vi "_Remote Prepare Run Data.vi"(4 "Ramp Parameters":T6[](array[typedef]), 5 "StepMass":dbl, 6 "# of Cycles":i32, 7 "StartMass":dbl, 8 "error in":errorcluster, 9 "Steps":i32, 10 "Pause (ms)":dbl, 11 "Dwell (ms)":dbl) -> (0 "error out":errorcluster, 3 "AcqMethod":T1[](array[typedef]) {"ScanType" format="%#.6g"; "Mass Range"."Res" items=["High/High", "Medium/Medium", "Low/Low", "High/Medium", "High/Low", "Medium/High", "Medium/Low", "Low/High", "Low/Medium"]})   [LabVIEW 2015]
uses:
  Type/_Ramp Parameter.ctl
  Type/_XML Expt.ctl
  Type/_XML Lens.ctl
  Type/_Mass Range Property.ctl
  Type/_Mass Range Parameters.ctl
  Type/_RT Res Type.ctl
  Type/_RT Parameter.ctl
  Type/_RT Active Ch.ctl
  Type/_RT Expt.ctl
  Type/_Run Mode.ctl
  Type/_RT Mass Range.ctl
  Type/_RT Command.ctl
  Configuration/_Global Configuration.vi
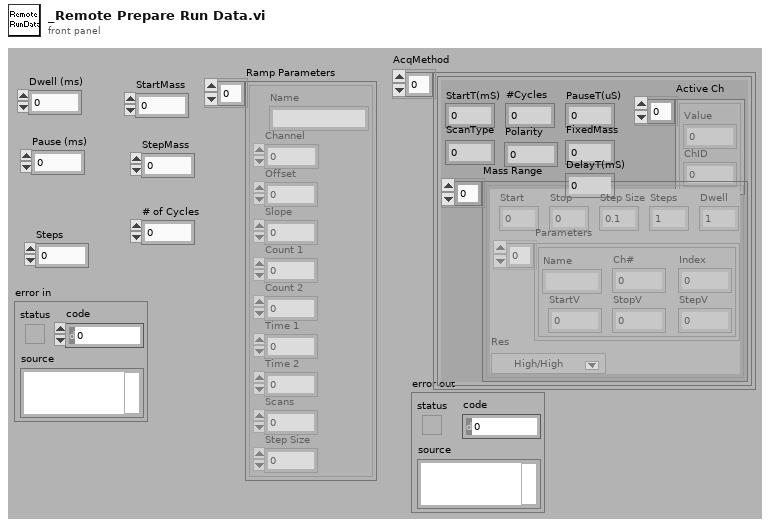
[diagram p1: front panel]
types:
  T1 = typedef "_XML Expt.ctl" = cluster{"StartT(mS)":i32, "#Cycles":i32, "PauseT(uS)":i32, "ScanType":i32, "Polarity":u8, "FixedMass":dbl, "DelayT(mS)":i32, "Active Ch":T2[], "Mass Range":T3[]}
  T2 = typedef "_XML Lens.ctl" = cluster{"Value":dbl, "ChID":u8}
  T3 = typedef "_Mass Range Property.ctl" = cluster{"Start":dbl, "Stop":dbl, "Step Size":dbl, "Steps":i32, "Dwell":dbl, "Parameters":T4[], "Res":T5}
  T4 = typedef "_Mass Range Parameters.ctl" = cluster{"Name":string, "Ch#":u8, "StartV":dbl, "StopV":dbl, "StepV":dbl, "Index":u8}
  T5 = typedef "_RT Res Type.ctl" = u16
  T6 = typedef "_Ramp Parameter.ctl" = cluster{"Name":string, "Channel":u8, "Offset":dbl, "Slope":dbl, "Count 1":dbl, "Count 2":dbl, "Time 1":dbl, "Time 2":dbl, "Scans":i32, "Step Size":dbl}
  T7 = typedef "_RT Command.ctl" = enum16{"xml Start Run", "xml Start Actual Run", "xml Stop Run", "xml Runtime Update", "xml Get Status", "xml Get Table", "xml Set Table", "xml Get Configuration", "xml System Status", "xml Set LC Input Logic", "xml Get Data", "xml Get Info", "Start", "StartActualRun", "Stop", "Runtime Update", "Get Data", "Get Info", "Get Status", "Get Param", "Get Config", "Get Table", "Read ADC", "Set Oscillator", "Update Config", "Update Table", "Set All Pol", "Set Pol and DC", "Set Max Mass", "Toggle RP", "Toggle EL", "Set PIC", "Initialize Turbo", "Send Turbo Comm", "Close Turbo", "P1", "P2", "P3", "Send Serial", "Set LC Out", "Get LC In", "Read VAC", "Test Table", "Toggle Power", "Get Startup", "Set Startup", "Get ADC Table", "Set ADC Table", "Get Brief Status", "Get Detail Status", "Auxiliary Update", "Set CC Logics", "Set CC Input Logics", "Ignore Error", "invalid"}
  T8 = typedef "_RT Mass Range.ctl" = cluster{"Steps":i32, "Dwell(uS)":i32, "Resolution Type":T5, "Ramping Ch":T9[]}
  T9 = typedef "_RT Active Ch.ctl" = cluster{"Start":i32, "Step":i32, "ChID":i32}
  T10 = typedef "_RT Expt.ctl" = cluster{"StartT(mS)":i32, "#Cycles":i32, "Scan Type":T11, "PauseT(uS)":i32, "Polarity":u8, "DelayT(mS)":i32, "Active Ch":T9[], "Mass Range":T8[]}
  T11 = typedef "_Run Mode.ctl" = enum16{"MRM (Q1/Q2)", "Q1 Scan", "Q1 SRM", "Q2 Scan", "Q2 SRM", "Product Scan", "Precursor Scan", "Neutral Loss", "Neutral Gain"}
  T12 = typedef "_RT Parameter.ctl" = cluster{"RunMode":i32, "Initial Ch":T9[], "Sync":u8, "Expt":T10[], "EqTime(mS)":i32}
  T13 = typedef "_Lens Property.ctl" = cluster{"Scan Type":u8, "Scans":i32, "Time 1":dbl, "Time 2":dbl, "Value 1":dbl, "Value 2":dbl, "Step Size":dbl}
  T14 = cluster{"Lenses":T13[], "Mass Ranges":T3[], "Acquire":bool, "MCA":bool, "Q1DC EN":bool, "Q1 POL":bool, "Q3 POL":bool, "Q1 RF  EN":bool, "Averaging":bool, "Log Scale":bool, "CPS":bool, "Unit":bool, "Data Path":path, "Run Mode":T11, "Fixed Mass (amu)":dbl, "Q3DC EN":bool, "Q3 RF  EN":bool, "Negative":bool}
  T15 = typedef "_RT Instrument 2.ctl" = cluster{"Table":T16[], "Instrument":string[]}
  T16 = typedef "_RT Configuration 2.ctl" = cluster{"Name":string, "Ch#":u8, "Min":dbl, "Max":dbl, "Def+":dbl, "Def-":dbl, "Offset":dbl, "Slope":dbl, "Type":u8, "Description":string, "SettleT":dbl}
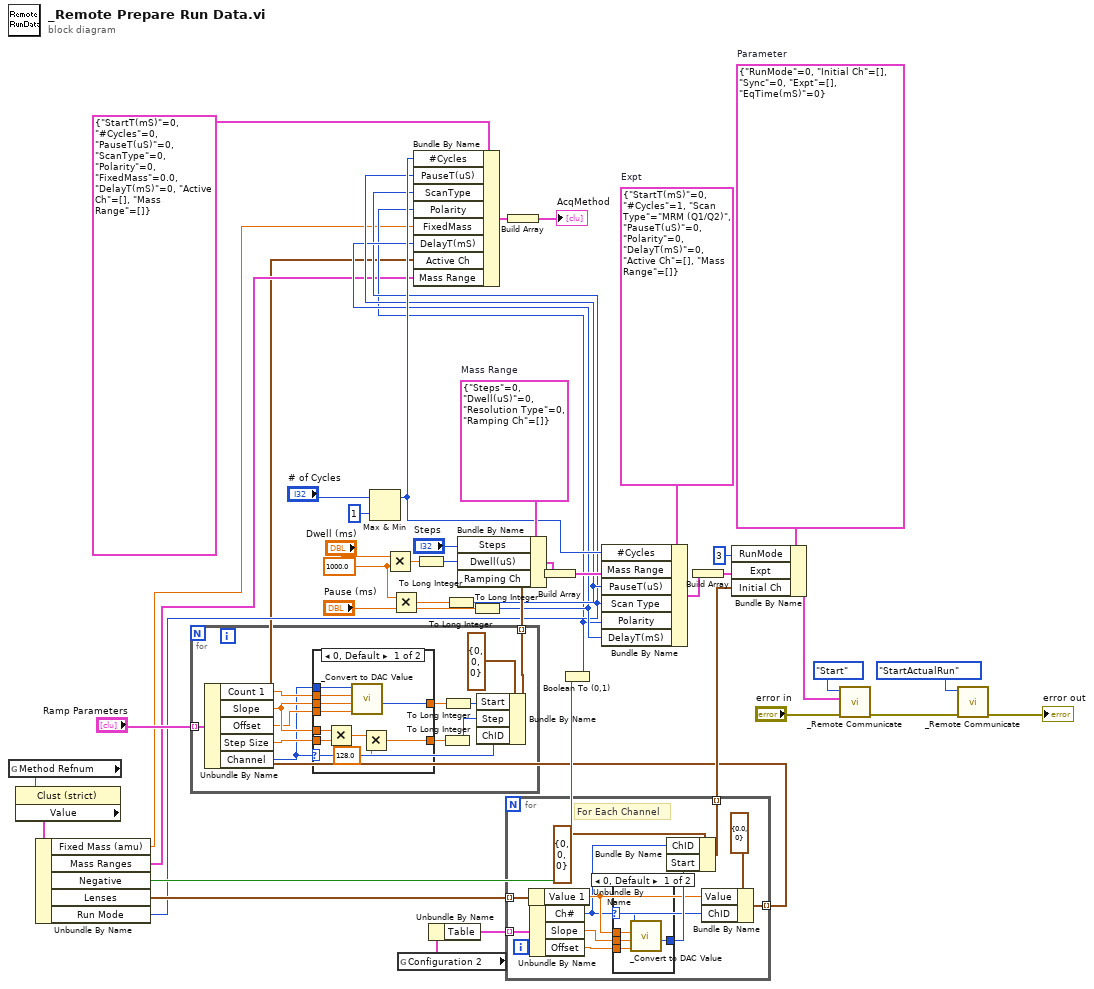
[diagram p0: block diagram]
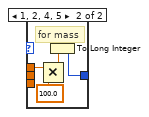
[diagram p2: hidden frame]
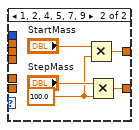
[diagram p3: hidden frame]
diagram:
  w33 = T8 {"Steps"=0, "Dwell(uS)"=0, "Resolution Type"=0, "Ramping Ch"=[]}  # Mass Range
  w37 = T10 {"StartT(mS)"=0, "#Cycles"=1, "Scan Type"=enum."MRM (Q1/Q2)", "PauseT(uS)"=0, "Polarity"=0, "DelayT(mS)"=0, "Active Ch"=[], "Mass Range"=[]}  # Expt
  w39 = T12 {"RunMode"=0, "Initial Ch"=[], "Sync"=0, "Expt"=[], "EqTime(mS)"=0}  # Parameter
  w27 = 1000.0 ("y")
  n1 = global read "_Global Configuration.vi" "Method Refnum"() -> (w24:refnum<vi>)
  n2 = property class="Clust (strict)"(reference=w24) -> ("Value"=w7:T14)  [unwired: 1 in, 2 out]
  n3 = Unbundle By Name(w7) -> ("Fixed Mass (amu)"=w6:dbl, "Mass Ranges"=w5:T3[], "Negative"=w17:bool, "Lenses"=w22:T13[], "Run Mode"=w9:T11)
  n4 = for {
    tunnel: "Ramp Parameters" -> [w55] mode=indexing
    tunnel: [w44] -> w28 mode=indexing
    n5 = Unbundle By Name(w55) -> ("Count 1"=w50:dbl, "Slope"=w49:dbl, "Offset"=w48:dbl, "Step Size"=w54:dbl, "Channel"=w45:u8)
    n6 = case shown="0, Default" w45 {
      tunnel: w54 -> [w64 _]
      tunnel: w49 -> [w65 _]
      tunnel: [w61 w69] -> w53
      tunnel: [w60 w66] -> w51
      tunnel: w45 -> [w59 _]
      tunnel: w50 -> [w58 _]
      tunnel: w49 -> [w57 _]
      tunnel: w48 -> [w56 _]
      frame 0, Default {
        n7 = Multiply(x=w65, y=w64) -> (x*y=w63:dbl)
        n8 = call "_Convert to DAC Value.vi"("Offset"=w56, "Slop"=w57, "Number"=w58, "Channel"=w59) -> ("DAC Value"=w60:i32)  [unwired: 1 in, 6 out]
        n9 = Multiply(x=w63, y=128.0) -> (x*y=w61:dbl)
      }
      frame 1, 2, 4, 5, 7, 9 {
        w67 = 100.0 ("y")
        n10 = Multiply(x="StartMass", y=w67) -> (x*y=w66:dbl)
        n11 = Multiply(x="StepMass", y=w67) -> (x*y=w69:dbl)
      }
    }
    n12 = To Long Integer(number=w53) -> (32bit integer=w46:i32)
    n13 = To Long Integer(number=w51) -> (32bit integer=w47:i32)
    n14 = Bundle By Name(cluster=T9 {"Start"=0, "Step"=0, "ChID"=0} ("Active Channel"), "Start"=w47, "Step"=w46, "ChID"=w45) -> (w44:T9)
  }
  n15 = Max & Min(x="# of Cycles", y=1) -> (max(x,y)=w12:i32)  [unwired: 1 out]
  n16 = Multiply(x="Dwell (ms)", y=w27) -> (x*y=w42:dbl)
  n17 = Multiply(x=w27, y="Pause (ms)") -> (x*y=w26:dbl)
  n18 = global read "_Global Configuration.vi" "Configuration 2"() -> (w23:T15)
  n19 = To Long Integer(number=w42) -> (32bit integer=w29:i32)
  n20 = Unbundle By Name(w23) -> ("Table"=w25:T16[])
  n21 = To Long Integer(number=w26) -> (32bit integer=w11:i32)
  n22 = Bundle By Name(cluster=w33, "Steps"="Steps", "Dwell(uS)"=w29, "Ramping Ch"=w28) -> (w32:T8)
  n23 = To Long Integer(number="Pause (ms)") -> (32bit integer=w10:i32)
  n24 = for {
    tunnel: [w77] -> w21 mode=indexing
    tunnel: w25 -> [w76] mode=indexing
    tunnel: w22 -> [w75] mode=indexing
    tunnel: [w71] -> w4 mode=indexing
    # "For Each Channel"
    n25 = Unbundle By Name(w75) -> ("Value 1"=w74:dbl)
    n26 = Unbundle By Name(w76) -> ("Ch#"=w73:u8, "Slope"=w81:dbl, "Offset"=w80:dbl)
    n27 = case shown="0, Default" w73 {
      selector: w73 -> [w82 _]
      tunnel: w74 -> [w86 w90]
      tunnel: w81 -> [w85 _]
      tunnel: w80 -> [w84 _]
      tunnel: [w83 w87] -> w78
      frame 0, Default {
        n28 = call "_Convert to DAC Value.vi"("Offset"=w84, "Slop"=w85, "Number"=w86, "Channel"=w82) -> ("DAC Value"=w83:i32)  [unwired: 2 in, 5 out]
      }
      frame 1, 2, 4, 5 {
        # "for mass"
        n29 = Multiply(x=w90, y=100.0) -> (x*y=w88:dbl)
        n30 = To Long Integer(number=w88) -> (32bit integer=w87:i32)
      }
    }
    n31 = Bundle By Name(cluster=T9 {"Start"=0, "Step"=0, "ChID"=0} ("Active Channel"), "ChID"=w73, "Start"=w78) -> (w77:T9)
    n32 = Bundle By Name(cluster=T2 {"Value"=0.0, "ChID"=0} ("Lens"), "Value"=w74, "ChID"=w73) -> (w71:T2)
  }
  n33 = Build Array(w32) -> (w31:T8[])
  n34 = Boolean To (0,1)(Boolean=w17) -> (0, 1=w8:i16)
  n35 = Bundle By Name(cluster=T1 {"StartT(mS)"=0, "#Cycles"=0, "PauseT(uS)"=0, "ScanType"=0, "Polarity"=0, "FixedMass"=0.0, "DelayT(mS)"=0, "Active Ch"=[], "Mass Range"=[]} ("Expt"), "#Cycles"=w12, "PauseT(uS)"=w11, "ScanType"=w9, "Polarity"=w8, "FixedMass"=w6, "DelayT(mS)"=w10, "Active Ch"=w4, "Mass Range"=w5) -> (w14:T1)
  n36 = Build Array(w14) -> (→"AcqMethod":T1[])
  n37 = Bundle By Name(cluster=w37, "#Cycles"=w12, "Mass Range"=w31, "PauseT(uS)"=w11, "Scan Type"=w9, "Polarity"=w8, "DelayT(mS)"=w10) -> (w36:T10)
  n38 = Build Array(w36) -> (w35:T10[])
  n39 = Bundle By Name(cluster=w39, "RunMode"=3, "Expt"=w35, "Initial Ch"=w21) -> (w34:T12)
  n40 = call "_Remote Communicate.vi"("error in (no error)"="error in", "Parameter"=w34, "Command"=_RT_Command."Start") -> ("error out"=w2:errorcluster)  [unwired: 3 in, 3 out]
  n41 = call "_Remote Communicate.vi"("error in (no error)"=w2, "Command"=_RT_Command."StartActualRun") -> ("error out"=→"error out":errorcluster)  [unwired: 4 in, 3 out]
